vi "NewRecord.vi"(8 "error in (no error)":errorcluster, 10 "Titles":string[](array[string])) -> (0 "error out":errorcluster, 3 "Record out":refnum<class "Record.lvclass">)   [LabVIEW 2015, in "Record.lvclass"]
uses:
  Record.lvclass
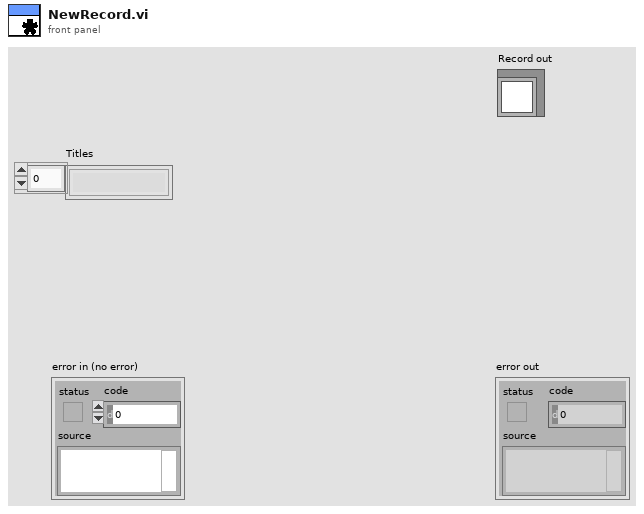
[diagram p1: front panel]
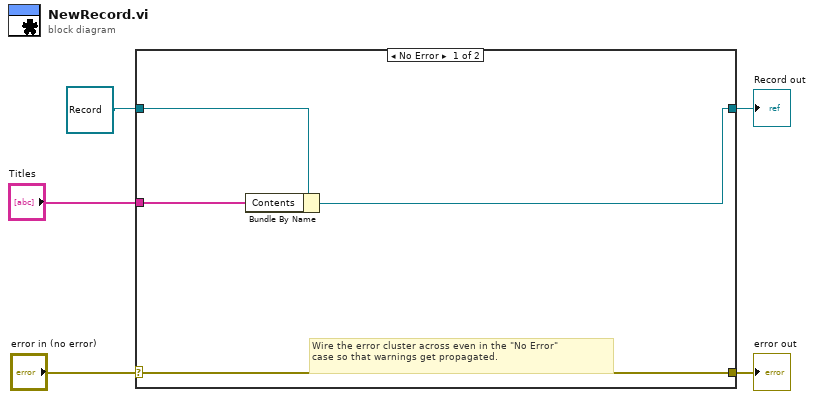
[diagram p0: block diagram]
diagram:
  n1 = case shown="No Error" "error in (no error)" {
    selector: "error in (no error)" -> [w9 w11]
    tunnel: [w9 w11] -> w4
    tunnel: [w6 w10] -> w2
    tunnel: refnum<class "Record.lvclass"> refnum ("Record in") -> [w8 w10]
    tunnel: "Titles" -> [w7 _]
    frame No Error {
      # "Wire the error cluster across even in the \"No Error\"\ncase so that warnings get propagated."
      n2 = Bundle By Name(cluster=w8, "Contents"=w7) -> (w6:refnum<class "Record.lvclass">)
    }
    frame Error {
    }
  }
  "error out" <- w4
  "Record out" <- w2
